vi "Log MTi.vi"(8 "error in (no error)":errorcluster, 11 "Vessel in":refnum<class "Vessel.lvclass">) -> (0 "error out":errorcluster, 3 "Vessel out":refnum<class "Vessel.lvclass">)   [LabVIEW 2014, in "Vessel.lvclass"]
uses:
  Vessel.lvclass
  <vilib>/imath/engines/lvmath/Plug In/_Char/NIMS_CH_character datatype.ctl
  <vilib>/imath/engines/lvmath2/RunTimeEngine/Managers/WorkSpace/UID Generator.vi
  <vilib>/imath/engines/lvmath/Plug In/_Char/NIMS_CH_String to Character Array.vi
  <vilib>/imath/engines/lvmath2/RunTimeEngine/BuiltInFunctions/length/NIMS_length(GV).vi
  <instcachedir>/0/NIMS_length(GV)_08A3D13377FD4E4B96F5795FBF3698FA.lvgen/NIMS_length(GV)_08A3D13377FD4E4B96F5795FBF3698FA_004.vi
  <vilib>/imath/engines/lvmath2/RunTimeEngine/RunTimeType/NIMS_RunTimeType_From StrictType (excl LVString).vi
  <instcachedir>/0/NIMS_RunTimeType_From StrictType (excl LVString)_15A5391EEA9C4AACB9955AC755B83D29.lvgen/NIMS_RunTimeType_From StrictType (excl LVString)_15A5391EEA9C4AACB9955AC755B83D29_000.vi
  <vilib>/imath/engines/lvmath2/RunTimeEngine/LocalVariableDefStatement/MC_LocalVariableDefStatement_Display.vi
  <vilib>/imath/engines/lvmath2/RunTimeEngine/RangeToken/NIMS_Range_R3 - Integer.vi
  <instcachedir>/0/NIMS_Range_R3 - Integer_66B9031982364693905FDE422E56E490.lvgen/NIMS_Range_R3 - Integer_66B9031982364693905FDE422E56E490_000.vi
  <vilib>/imath/engines/lvmath2/RunTimeEngine/CommandStatement/MC_CommandStatement_break.vi
  <vilib>/imath/engines/lvmath/Plug In/_Char/NIMS_CH_Character 2D to String 1D.vi
  <vilib>/imath/engines/lvmath2/RunTimeEngine/IndexRead/NIMS V(S).vi
  <instcachedir>/0/NIMS V(S)_0488751826AF41519A22953C041130DC.lvgen/NIMS V(S)_0488751826AF41519A22953C041130DC_003.vi
  <vilib>/imath/engines/lvmath2/RunTimeEngine/BuiltInFunctions/strcmp/NIMS_strcmp.vi
  <vilib>/imathl/engines/lvmath/Functions/Error Handling/Create Error.vi
  <vilib>/imath/engines/lvmath2/RunTimeEngine/VariableToken/NIMS_VariableToken_CondDefined.vi
  <instcachedir>/0/NIMS_VariableToken_CondDefined_EE8DD211A89249938CE6537267F5C9B3.lvgen/NIMS_VariableToken_CondDefined_EE8DD211A89249938CE6537267F5C9B3_003.vi
  <vilib>/imath/engines/lvmath2/RunTimeEngine/Managers/SymbolTable/Clear UID.vi
  <vilib>/imath/engines/lvmath2/RunTimeEngine/NodeEndStatement/NIMS_NodeEndStatement_Output.vi
  <instcachedir>/0/NIMS_NodeEndStatement_Output_53EC0D466D134D7ABD903AC30B43404B.lvgen/NIMS_NodeEndStatement_Output_53EC0D466D134D7ABD903AC30B43404B_011.vi
  <vilib>/imath/engines/lvmath2/RunTimeEngine/ErrorHandling/NIMS_Finalize Error.vi
  <vilib>/imath/engines/lvmath2/RunTimeEngine/IndexRead/NIMS V(R2).vi
  <instcachedir>/0/NIMS V(R2)_C76619605A0E4E9F8B2FA9389712AC47.lvgen/NIMS V(R2)_C76619605A0E4E9F8B2FA9389712AC47_002.vi
  <vilib>/imath/engines/lvmath/Plug In/_Char/NIMS_CH_Character RV to String.vi
  <instcachedir>/0/NIMS_NodeEndStatement_Output_53EC0D466D134D7ABD903AC30B43404B.lvgen/NIMS_NodeEndStatement_Output_53EC0D466D134D7ABD903AC30B43404B_009.vi
  Supervisor/Supervisor.lvclass
  <vilib>/imath/engines/lvmath2/RunTimeEngine/Managers/SymbolTable/NIMS_WorkSpace.lvlib
panel:
  out "path to log files":string
  out "path 2":path
  out "path":path
  out "log line raw":string="21:11:09.2343\t-0.00\t0.00\t30.00\t0.00\t0.00\t-0.00\t0.00\t0.01\t-0.01\t-0.00\t30.00\t0.00\t0.00\t-0.00\t0.00\t0.00\t0.00\t0.00\t30.00\t0.00\t0.00\t0.00\t0.00\t0.00\t132.54\t-43.98\t11.70\t-0.09\t-661 \t252 \t818 \t705 \r\n"
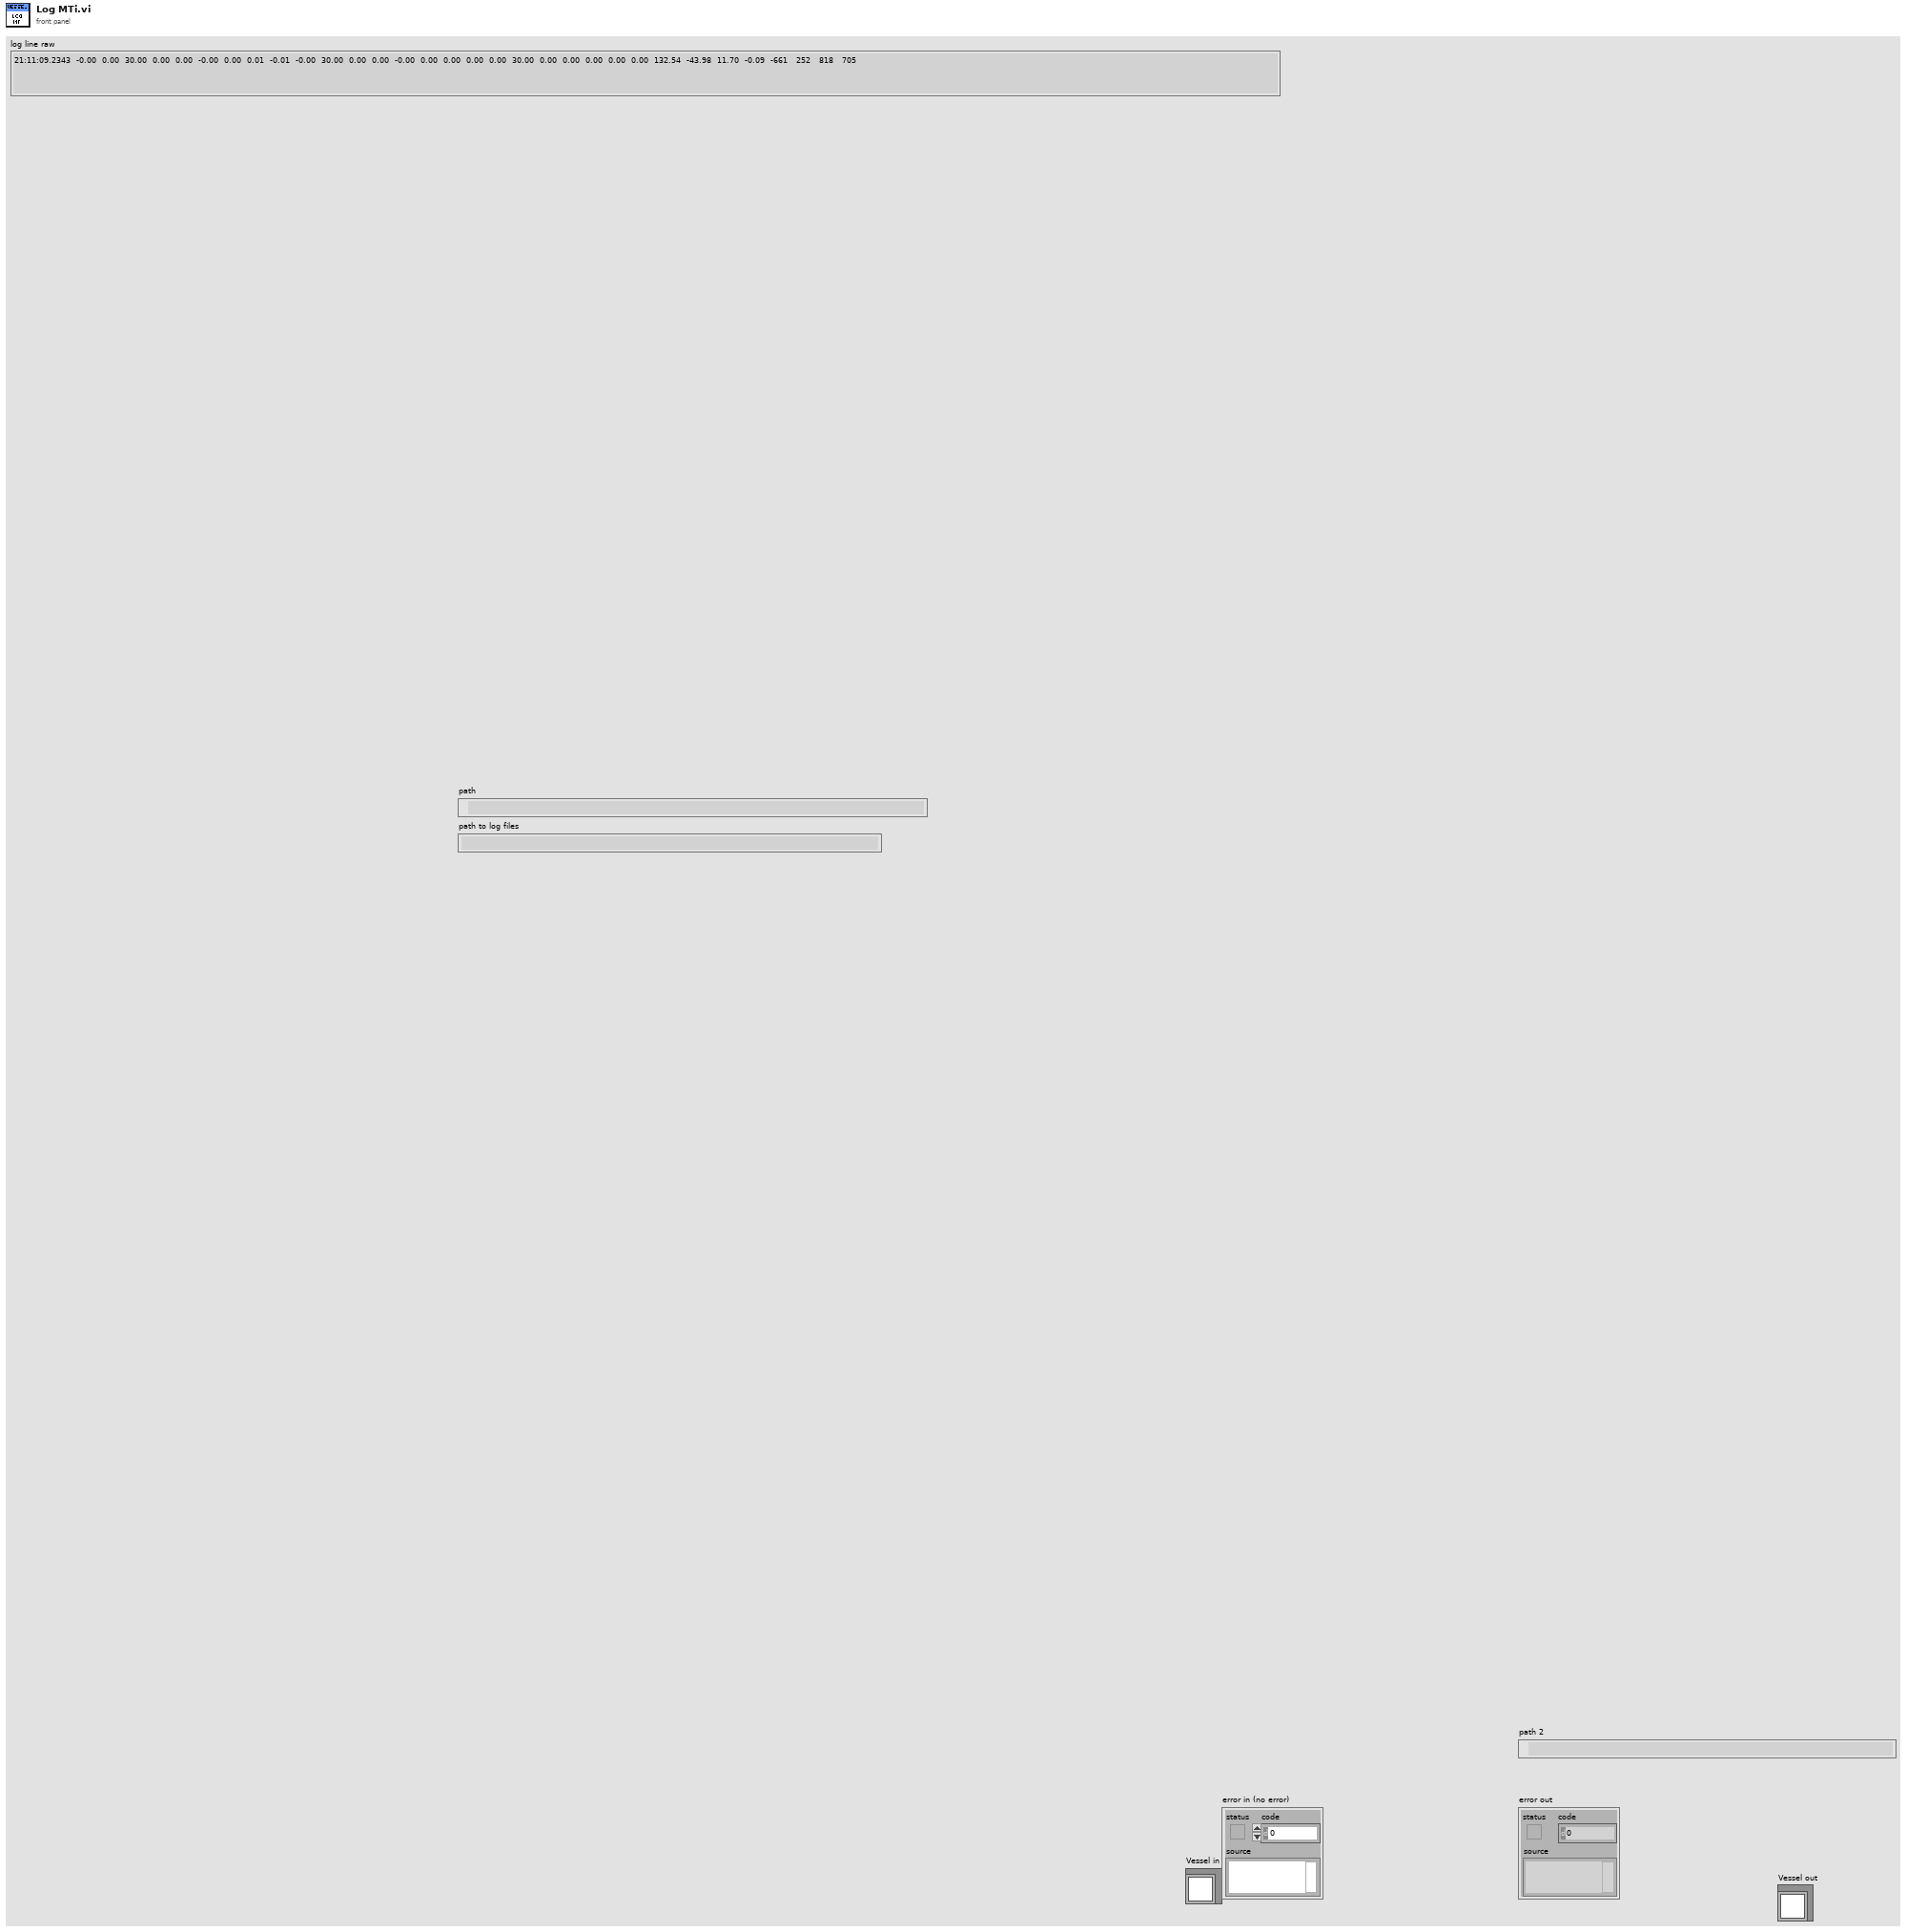
[diagram p1: front panel]
types:
  T1 = typedef "NIMS_CH_character datatype.ctl" = cluster{"Numeric":u8}
  T2 = enum16{"open", "replace", "create", "open or create", "replace or create", "replace or create with confirmation"}
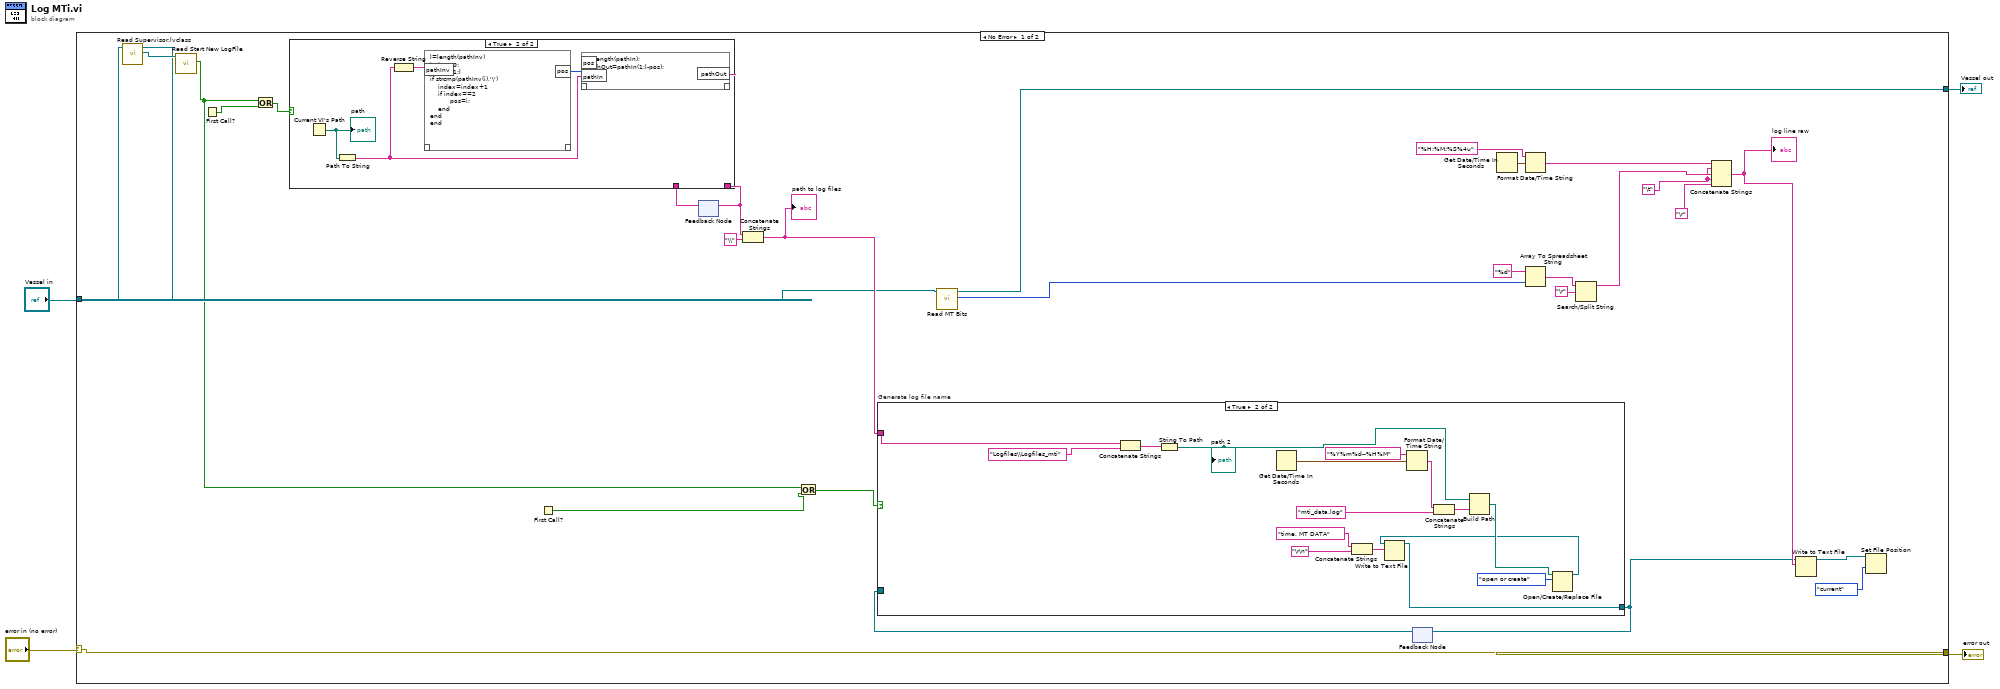
[diagram p0: block diagram]
diagram:
  n1 = case shown="No Error" "error in (no error)" {
    selector: "error in (no error)" -> [w21 w279]
    tunnel: [w21 w279] -> w1
    tunnel: [w15 w278] -> w3
    tunnel: "Vessel in" -> [w13 w278]
    frame No Error {
      w22 = "\t"
      n2 = call "Read Supervisor.lvclass.vi"("Vessel in"=w13) -> ("Supervisor.lvclass"=w14:refnum<class "Supervisor.lvclass">, "Vessel out"=w12:refnum<class "Vessel.lvclass">)  [unwired: 8 in, 1 out]
      n3 = call-dynamic "Read Start New LogFile.vi"("Supervisor in"=w14) -> ("Start New LogFile"=w8:bool)  [unwired: 8 in, 2 out]
      n4 = First Call?() -> (First Call?: T/F=w11:bool)
      n5 = Or(x=w8, y=w11) -> (x .or. y?=w10:bool)
      n6 = First Call?() -> (First Call?: T/F=w9:bool)
      n7 = feedback #1() -> (w19:string)  [unwired: 1 in]
      n8 = case shown="True" w10 {
        tunnel: [w34 w35] -> w18
        tunnel: w19 -> [w34 _]
        frame False {
        }
        frame True {
          n9 = Current VI's Path() -> (path=w39:path)
          "path" <- w39
          n10 = Path To String(path=w39) -> (string=w37:string)
          n11 = Reverse String(1:w37) -> (0:w38:string)
          n12 = mathscript code="l=length(pathInv)\nindex=0;\nfor i=1:1:l\nif strcmp(pathInv(i),'\\')\n    index=index+1\n    if index==2\n          pos=i;\n    end\nend\nend"("pathInv"=w38) -> ("pos"=w36:i32)  [unwired: 1 in, 1 out]
          n13 = mathscript code="l=length(pathIn);\npathOut=pathIn(1:l-pos);"("pathIn"=w37, "pos"=w36) -> ("pathOut"=w35:string)  [unwired: 1 in, 1 out]
        }
      }
      n14 = feedback-in #1(w18) -> ()
      n15 = Concatenate Strings(w18, "\\" ("string")) -> (w16:string)
      "path to log files" <- w16
      n16 = Or(x=w8, y=w9) -> (x .or. y?=w7:bool)
      n17 = call-dynamic "Read MT Bits.vi"("Vessel in"=w12) -> ("MT Bits"=w20:u8[], "Vessel out"=w15:refnum<class "Vessel.lvclass">)  [unwired: 8 in, 1 out]
      n18 = feedback #2() -> (w6:refnum<file>)  [unwired: 1 in]
      n19 = case "Generate log file name" shown="True" w7 {
        tunnel: [w261 w266] -> w5
        tunnel: w16 -> [_ w264]
        tunnel: w6 -> [w261 _]
        frame False {
        }
        frame True {
          n20 = Concatenate Strings(w264, "Logfiles\\Logfiles_mti" ("string")) -> (w263:string)
          n21 = String To Path(string=w263) -> (path=w262:path)
          "path 2" <- w262
          n22 = Get Date/Time In Seconds() -> (seconds since 1Jan1904=w274:timestamp)
          n23 = Concatenate Strings("time, MT DATA" ("string"), "\r\n") -> (w268:string)
          n24 = Format Date/Time String(time format string (%c)="%Y%m%d--%H%M", seconds (now)=w274) -> (date/time string=w272:string)  [unwired: 1 in]
          n25 = Concatenate Strings(w272, "mti_data.log" ("string")) -> (w276:string)
          n26 = Build Path(base path=w262, name or relative path=w276) -> (appended path=w275:path)
          n27 = Open/Create/Replace File(file path (use dialog)=w275, operation (0:open)=T2."open or create") -> (refnum out=w267:refnum<file>)  [unwired: 4 in, 2 out]
          n28 = Write to Text File(file (use dialog)=w267, text=w268) -> (refnum out=w266:refnum<file>)  [unwired: 2 in, 2 out]
        }
      }
      n29 = feedback-in #2(w5) -> ()
      n30 = Get Date/Time In Seconds() -> (seconds since 1Jan1904=w30:timestamp)
      n31 = Format Date/Time String(time format string (%c)="%H:%M:%S%4u", seconds (now)=w30) -> (date/time string=w24:string)  [unwired: 1 in]
      n32 = Array To Spreadsheet String(array=w20, 3:"%d" ("format string")) -> (spreadsheet string=w25:string)  [unwired: 1 in]
      n33 = Search/Split String(string=w25, search string/char (-)="\r") -> (substring before match=w32:string)  [unwired: 1 in, 2 out]
      n34 = Concatenate Strings(w24, w22, w32, w22, "\r") -> (w27:string)
      "log line raw" <- w27
      n35 = Write to Text File(file (use dialog)=w5, text=w27) -> (refnum out=w29:refnum<file>)  [unwired: 2 in, 2 out]
      n36 = Set File Position(refnum=w29, from (0:start)=enum16{"start", "end", "current"}."current") -> ()  [unwired: 2 in, 2 out]
    }
    frame Error {
    }
  }
  "Vessel out" <- w3
  "error out" <- w1
